vi "Measurement UI.vi"() -> ()   [LabVIEW 2021, in "start-up UI.lvlib"]
uses:
  start-up UI.lvlib
panel:
  in  "Meas Graphs":enum32{"LED V-I Characteristics"}(tab)
  out "LEDInputGraph":cluster{"Value":dbl[], "Value":dbl[]}(graph)
  out "LEDOutputGraph":cluster{dbl[], dbl[]}(graph)
  in  "MeasConfigurations":T1(tab)=enum."Source Config"
  in  "LED current (Io)":dbl=1.0 caption="OUTPUT CURRENT (Io)" format="%.3pA"
  in  "Cumulative forward voltage (Vf)":dbl=1.0 caption="FORWARD VOLTAGE (Vf)" format="%.3fV"
  in  "LED voltage (Vo)":dbl=1.0 caption="OUTPUT VOLTAGE (Vo)" format="%.3fV"
  in  "Source delay":dbl=0.005 caption="SOURCE DELAY" format="%.3ps"
  in  "DUT setup time":dbl=1.0 caption="DUT SETUP TIME" format="%.3ps"
  in  "Aperture time":dbl=0.005 caption="APERTURE TIME" format="%.3ps"
  in  "Source current limit":dbl=14.0 caption="CURRENT LIMIT" format="%#_6pA"
  in  "PPSResourceName":refnum<k15> caption="RESOURCE NAME"
  in  "Source stop voltage":dbl=14.0 caption="VOLTAGE STOP LEVEL" format="%#_6pV"
  in  "Source sense":i32(ring)=1009 caption="SENSE" items=["Local"=1008, "Remote"=1009]
  in  "Source maximum power":dbl=20.0 caption="MAXIMUM POWER" format="%#_6pW"
  in  "Source start voltage":dbl=6.0 caption="VOLTAGE START LEVEL" format="%#_6pV"
  in  "Source voltage sweep points":i32=4 caption="NO. OF POINTS"
  in  "DUT current limit":dbl=6.0 caption="DUT CURRENT LIMIT" format="%#_6pA"
  in  "Load current range":string(combo) caption="CURRENT LIMIT RANGE"
  in  "Load voltage limit":dbl caption="VOLTAGE  LIMIT" format="%#_6pV"
  in  "Load voltage level range":dbl=6.0 caption="VOLTAGE LEVEL RANGE" format="%#_6pV"
  in  "Load sense":i32(ring)=1009 caption="SENSE" items=["Local"=1008, "Remote"=1009]
  in  "LoadResourceName":refnum<k15> caption="RESOURCE NAME"
  out "Status":string
  in  "Max output resistance":string caption="RESOURCE NAME"
  in  "Load current limit range":string caption="RESOURCE NAME"
  out "Load current":dbl[](array[numeric])
  out "Source current":dbl[](array[numeric])
  out "Load voltages":dbl[](array[numeric])
  out "Source voltages":dbl[](array[numeric])
  in  "Source resource name":string caption="RESOURCE NAME"
  in  "Load resource name":string caption="RESOURCE NAME"
  # "V(in) vs I(in)"
  # "Iin vs Vin"
  # "Iout vs Vout"
  # "Emulated LED Configuration"
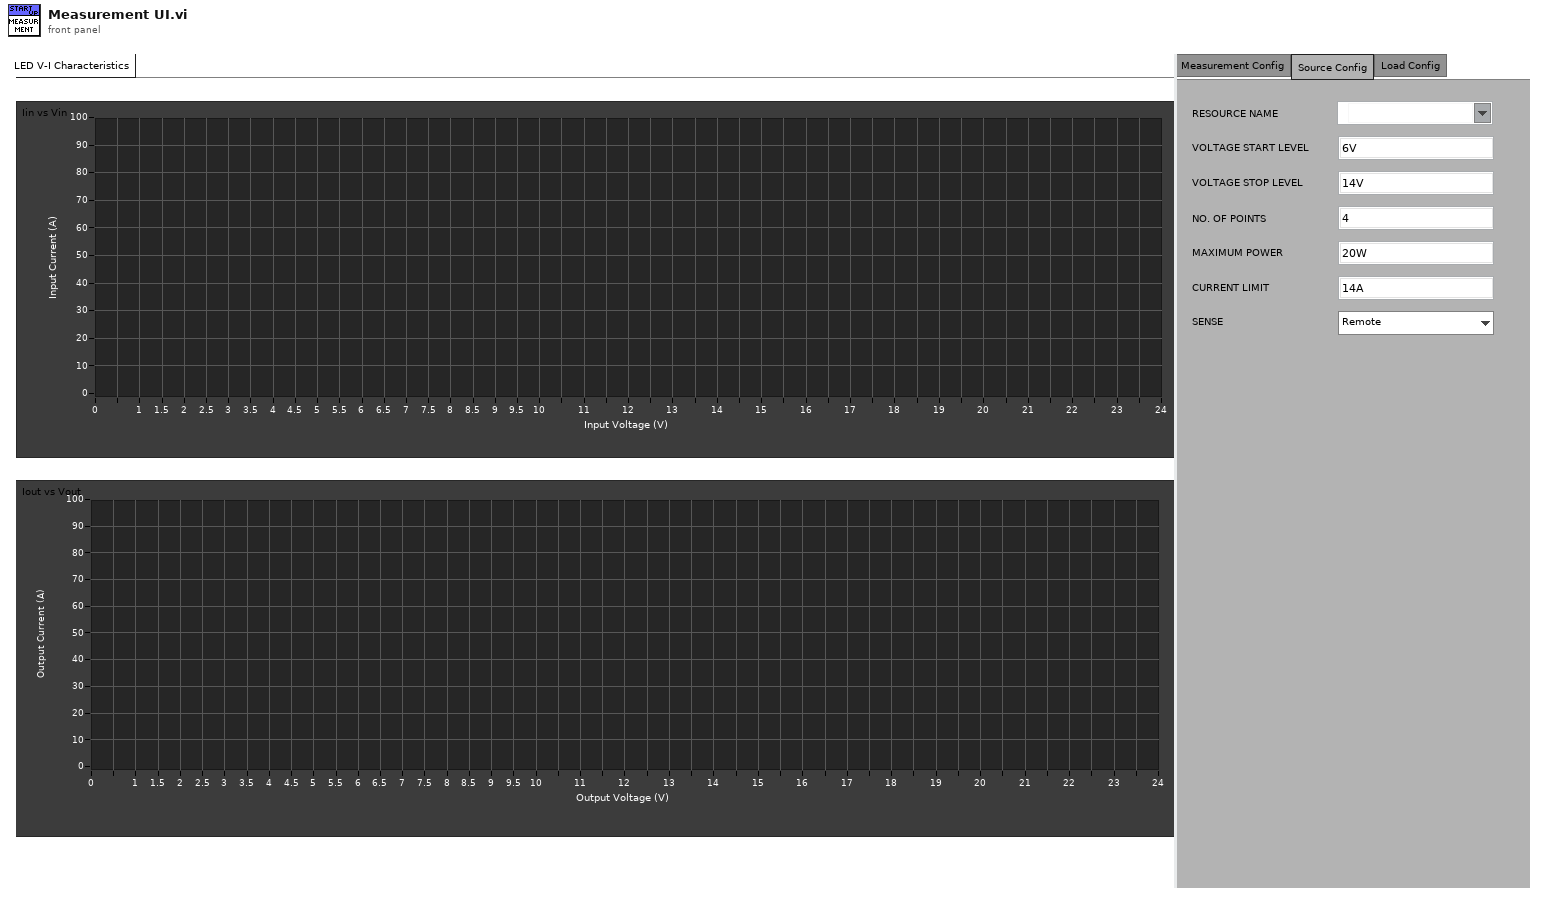
[diagram p1: front panel]
types:
  T1 = enum32{"Measurement Config", "Source Config", "Load Config", "Hidden Controls"}
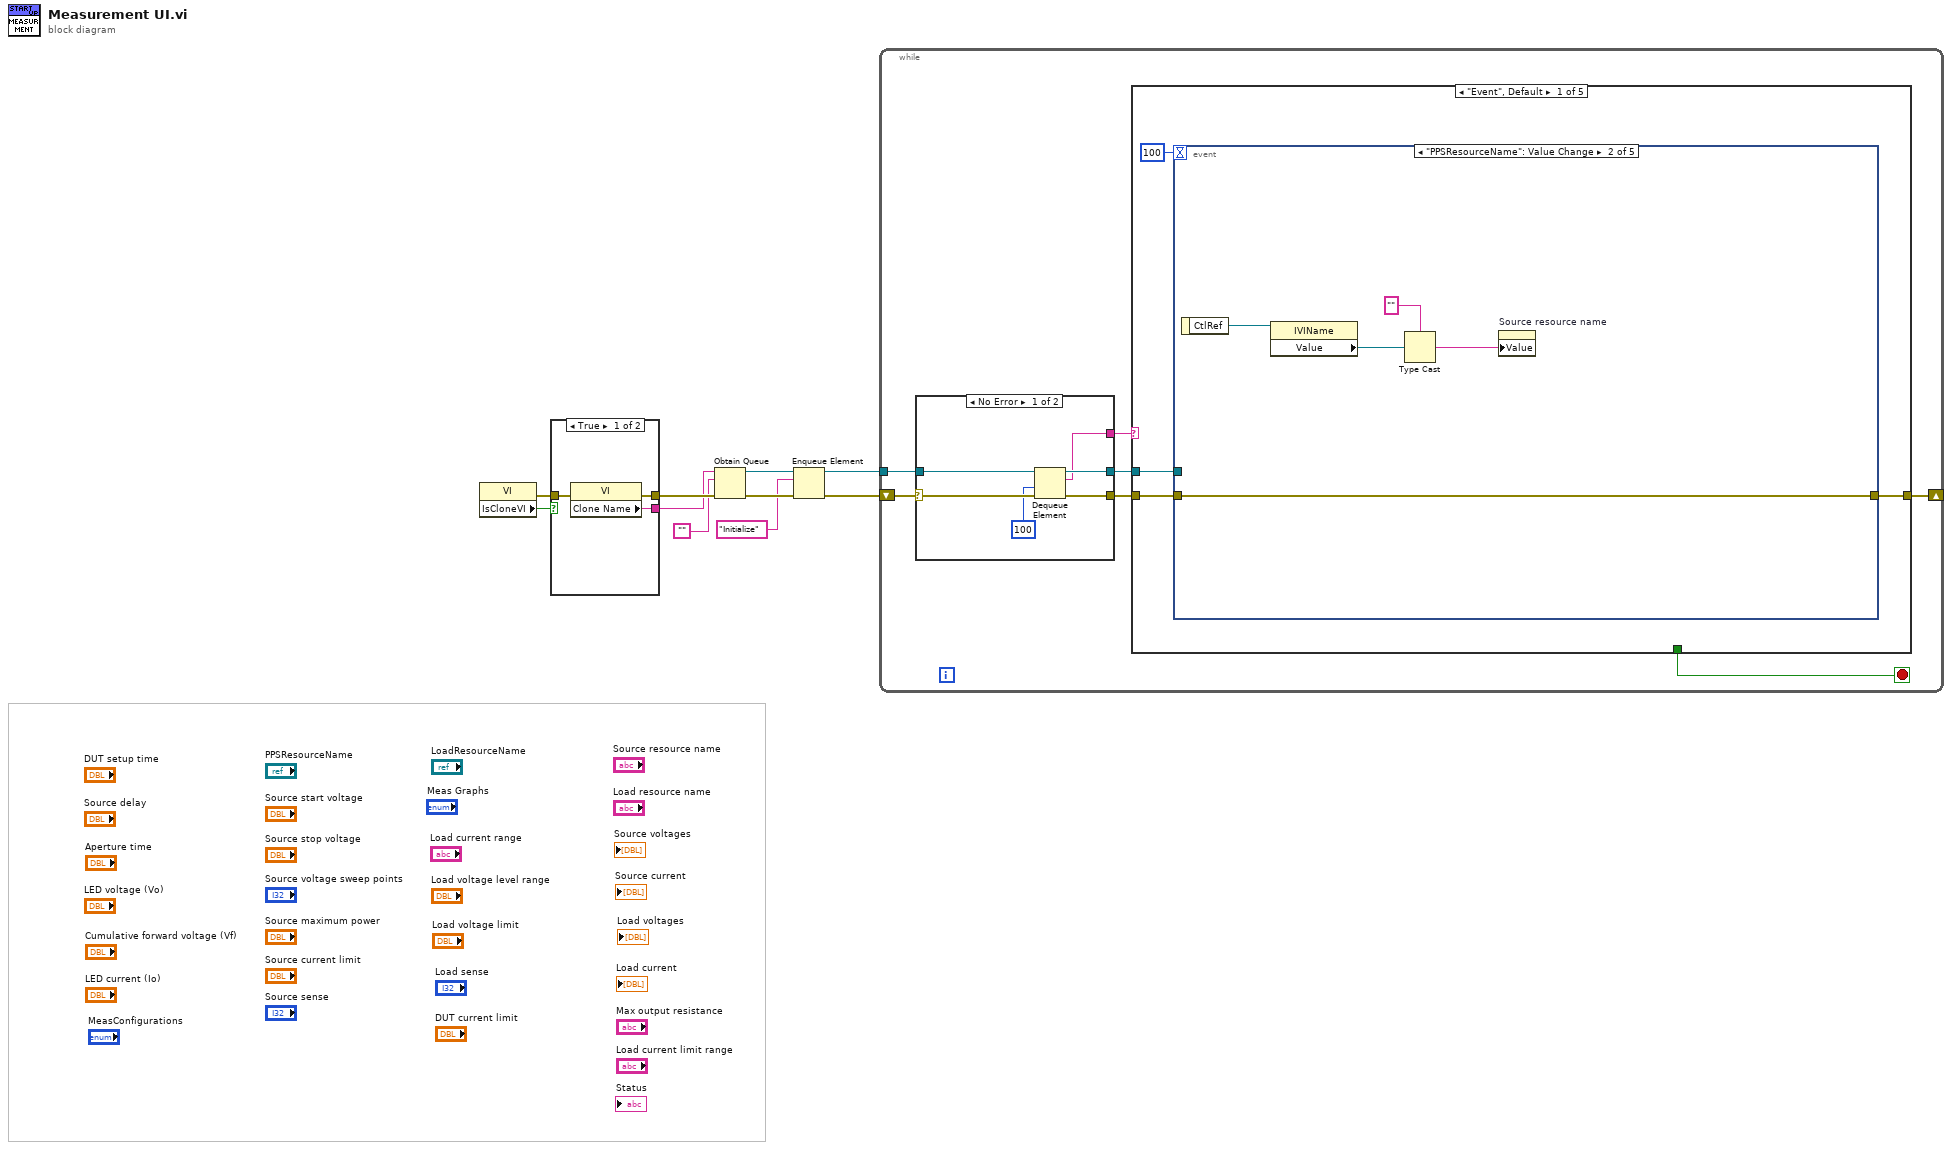
[diagram p0: block diagram]
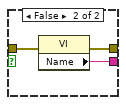
[diagram p2: hidden frame]
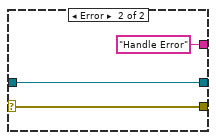
[diagram p3: hidden frame]
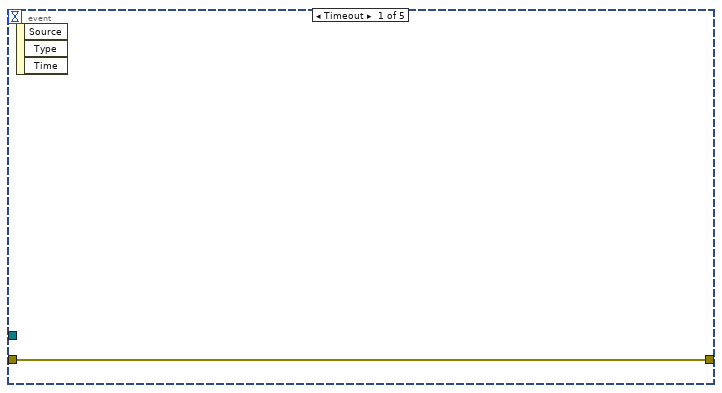
[diagram p4: hidden frame]
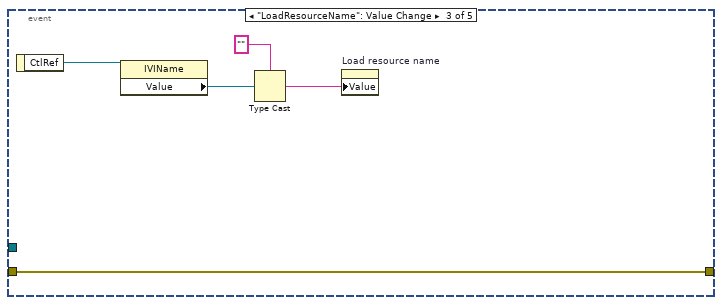
[diagram p5: hidden frame]
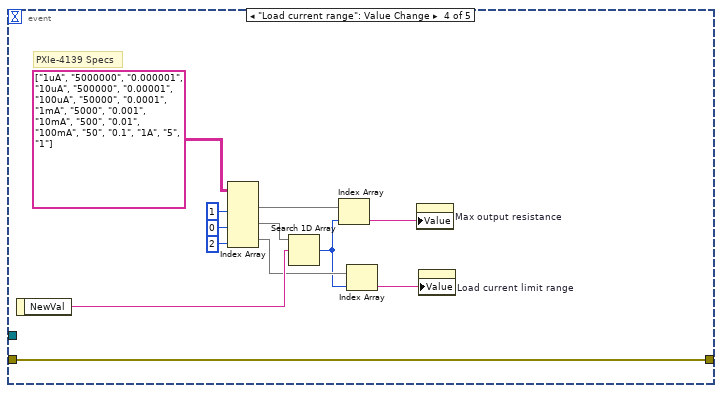
[diagram p6: hidden frame]
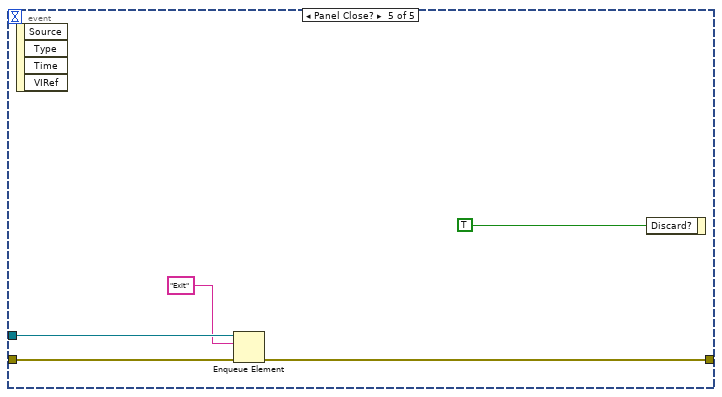
[diagram p7: hidden frame]
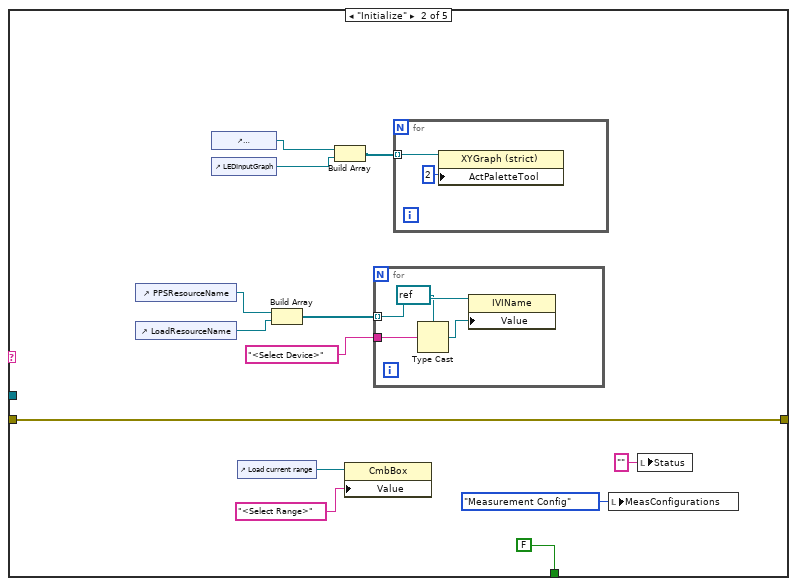
[diagram p8: hidden frame]
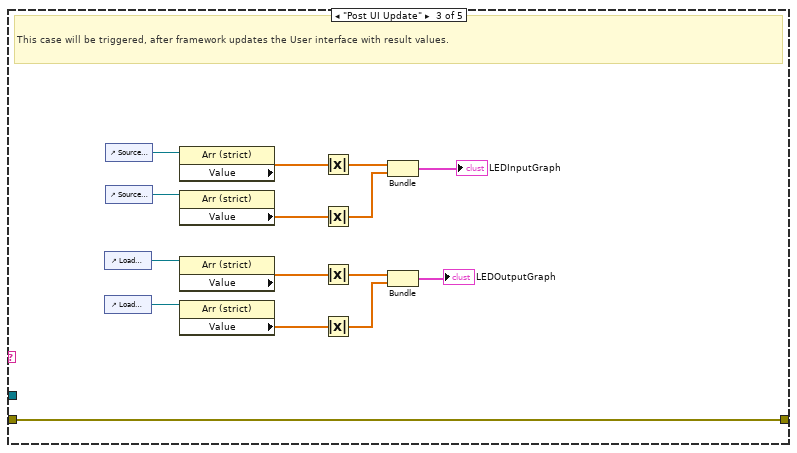
[diagram p9: hidden frame]
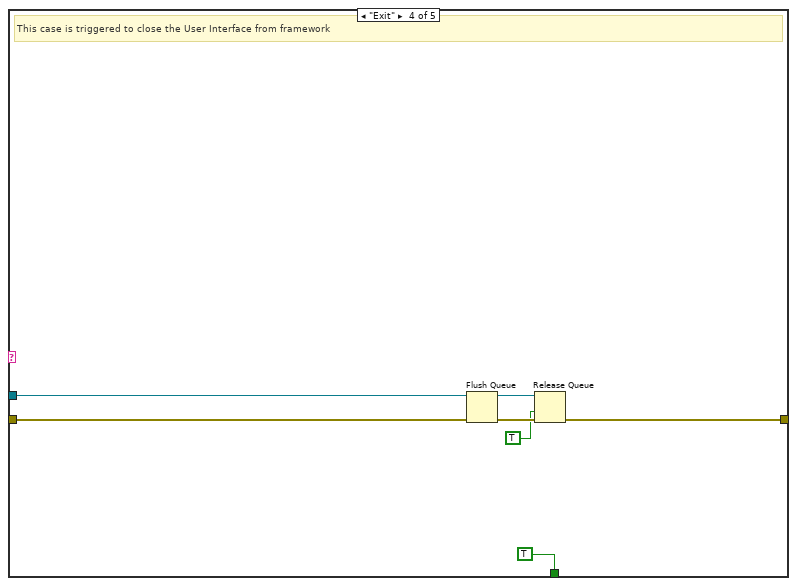
[diagram p10: hidden frame]
diagram:
  n1 = property class="VI"() -> (error out=w1:errorcluster, "IsCloneVI"=w2:bool)  [unwired: 2 in, 1 out]
  n2 = case shown="True" w2 {
    tunnel: [w13 w16] -> w10
    tunnel: [w12 w15] -> w9
    tunnel: w1 -> [w11 w14]
    frame True {
      n3 = property class="VI"(error in=w11) -> (error out=w13:errorcluster, "Clone Name"=w12:string)  [unwired: 1 in, 1 out]
    }
    frame False {
      n4 = property class="VI"(error in=w14) -> (error out=w16:errorcluster, "Name"=w15:string)  [unwired: 1 in, 1 out]
    }
  }
  n5 = Obtain Queue(name (unnamed)=w9, element data type="", error in (no error)=w10) -> (queue out=w6:refnum<queue>, error out=w8:errorcluster)  [unwired: 2 in, 1 out]
  n6 = Enqueue Element(queue=w6, element="Initialize", error in (no error)=w8) -> (queue out=w5:refnum<queue>, error out=w7:errorcluster)  [unwired: 1 in, 1 out]
  n7 = while {
    shift-right: [w18] -> _
    shift-left: w7 -> [w23]
    tunnel: w5 -> [w21]
    stop <- w17 stop-if-true
    n8 = case shown="No Error" w23 {
      selector: w23 -> [w29 w32]
      tunnel: [w28 w32] -> w22
      tunnel: w21 -> [w27 w31]
      tunnel: [w26 w31] -> w20
      tunnel: [w25 "Handle Error"] -> w19
      frame No Error {
        n9 = Dequeue Element(queue=w27, timeout in ms (-1)=100, error in (no error)=w29) -> (queue out=w26:refnum<queue>, element=w25:string, error out=w28:errorcluster)  [unwired: 1 out]
      }
      frame Error {
      }
    }
    n10 = case shown="\"Event\", Default" w19 {
      tunnel: w22 -> [w35 w77 w98 w105 w106]
      tunnel: w20 -> [w33 _ _ w103 _]
      tunnel: [w36 w77 w98 w100 w106] -> w18
      tunnel: [_ FALSE _ TRUE _] -> w17
      frame "Event", Default {
        n11 = event shown="[1] \"PPSResourceName\": Value Change" {
          selector: _ -> [_ _ _ _ _]
          dyn-events: _ -> [_ _ _ _ _]
          timeout: 100 -> [_ _ _ _ _]
          tunnel: [w37 w38 w43 w54 w62] -> w36
          tunnel: w35 -> [w37 w38 w43 w54 w63]
          tunnel: w33 -> [_ _ _ _ w61]
          event Timeout {
            n12 = event-data() -> ()  [unwired: 1 in, 3 out]
          }
          event "PPSResourceName": Value Change {
            n13 = event-data() -> ("CtlRef"=w42:refnum<vi>)  [unwired: 1 in]
            n14 = property class="IVIName"(reference=w42) -> ("Value"=w40:refnum<k15>)  [unwired: 1 in, 2 out]
            n15 = Type Cast(type="", x=w40) -> (*(type *) &x=w41:string)
            n16 = property on="Source resource name" class="Str"("Value"=w41) -> ()  [unwired: 2 in, 2 out]
          }
          event "LoadResourceName": Value Change {
            n17 = event-data() -> ("CtlRef"=w45:refnum<vi>)  [unwired: 1 in]
            n18 = property class="IVIName"(reference=w45) -> ("Value"=w47:refnum<k15>)  [unwired: 1 in, 2 out]
            n19 = Type Cast(type="", x=w47) -> (*(type *) &x=w44:string)
            n20 = property on="Load resource name" class="Str"("Value"=w44) -> ()  [unwired: 2 in, 2 out]
          }
          event "Load current range": Value Change {
            # "PXIe-4139 Specs"
            n21 = event-data() -> ("NewVal"=w57:string)  [unwired: 1 in]
            n22 = Index Array(array=string[][] [["1uA", "5000000", "0.000001"], ["10uA", "500000", "0.00001"], ["100uA", "50000", "0.0001"], ["1mA", "5000", "0.001"], ["10mA", "500", "0.01"], ["100mA", "50", "0.1"], ["1A", "5", "1"]], index (col) #1=1 ("disabled index (col)"), index (col) #2=0 ("index (col)"), index (col) #3=2 ("index (col)")) -> (element #1=w55:string[], element #2=w50:string[], element #3=w51:string[])  [unwired: 3 in]
            n23 = Search 1D Array(1D array=w50, element=w57) -> (index of element=w49:i32)  [unwired: 1 in]
            n24 = Index Array(array=w55, index=w49) -> (element=w53:string)
            n25 = Index Array(array=w51, index=w49) -> (element=w48:string)
            n26 = property on="Max output resistance" class="Str"("Value"=w53) -> ()  [unwired: 2 in, 2 out]
            n27 = property on="Load current limit range" class="Str"("Value"=w48) -> ()  [unwired: 2 in, 2 out]
          }
          event Panel Close? {
            n28 = event-data() -> ()  [unwired: 1 in, 4 out]
            n29 = Enqueue Element(queue=w61, element="Exit", error in (no error)=w63) -> (error out=w62:errorcluster)  [unwired: 1 in, 2 out]
            n30 = event-data("Discard?"=TRUE) -> ()  [unwired: 1 in, 1 out]
          }
        }
      }
      frame "Initialize" {
        n31 = control-ref of="PPSResourceName"() -> (w72:refnum<vi>)
        n32 = control-ref of="LoadResourceName"() -> (w71:refnum<vi>)
        n33 = control-ref of="LEDOutputGraph"() -> (w74:refnum<vi>)
        n34 = control-ref of="LEDInputGraph"() -> (w73:refnum<vi>)
        n35 = control-ref of="Load current range"() -> (w68:refnum<vi>)
        n36 = Build Array(w72, w71) -> (w70:refnum<vi>[])
        n37 = Build Array(w74, w73) -> (w75:refnum<vi>[])
        n38 = property class="CmbBox"(reference=w68, "Value"="<Select Range>") -> ()  [unwired: 1 in, 2 out]
        n39 = for {
          tunnel: w70 -> [w81] mode=indexing
          tunnel: "<Select Device>" -> [w80]
          n40 = Type Cast(type=refnum<k15> refnum ("Value"), x=w80) -> (*(type *) &x=w78:refnum<k15>)
          n41 = property class="IVIName"(reference=w81, "Value"=w78) -> ()  [unwired: 1 in, 2 out]
        }
        n42 = for {
          tunnel: w75 -> [w82] mode=indexing
          n43 = property class="XYGraph (strict)"(reference=w82, "ActPaletteTool"=2 ("Palette:Active Tool")) -> ()  [unwired: 1 in, 2 out]
        }
        n44 = local write "MeasConfigurations"(T1."Measurement Config" ("MeasConfigurations")) -> ()
        n45 = local write "Status"("" ("Status")) -> ()
      }
      frame "Post UI Update" {
        # "This case will be triggered, after framework updates the User interface with result values."
        n46 = control-ref of="Load voltages"() -> (w87:refnum<vi>)
        n47 = control-ref of="Load current"() -> (w86:refnum<vi>)
        n48 = control-ref of="Source voltages"() -> (w97:refnum<vi>)
        n49 = control-ref of="Source current"() -> (w96:refnum<vi>)
        n50 = property class="Arr (strict)"(reference=w97) -> ("Value"=w95:dbl[])  [unwired: 1 in, 2 out]
        n51 = property class="Arr (strict)"(reference=w96) -> ("Value"=w94:dbl[])  [unwired: 1 in, 2 out]
        n52 = property class="Arr (strict)"(reference=w87) -> ("Value"=w88:dbl[])  [unwired: 1 in, 2 out]
        n53 = property class="Arr (strict)"(reference=w86) -> ("Value"=w89:dbl[])  [unwired: 1 in, 2 out]
        n54 = Absolute Value(x=w95) -> (abs(x)=w93:dbl[])
        n55 = Absolute Value(x=w94) -> (abs(x)=w92:dbl[])
        n56 = Absolute Value(x=w88) -> (abs(x)=w90:dbl[])
        n57 = Absolute Value(x=w89) -> (abs(x)=w91:dbl[])
        n58 = Bundle(w93, w92) -> (→"LEDInputGraph":cluster{dbl[], dbl[]})  [unwired: 1 in]
        n59 = Bundle(w90, w91) -> (→"LEDOutputGraph":cluster{dbl[], dbl[]})  [unwired: 1 in]
      }
      frame "Exit" {
        # "This case is triggered to close the User Interface from framework"
        n60 = Flush Queue(queue=w103, error in (no error)=w105) -> (queue out=w102:refnum<queue>, error out=w101:errorcluster)  [unwired: 1 out]
        n61 = Release Queue(queue=w102, force destroy? (F)=TRUE, error in (no error)=w101) -> (error out=w100:errorcluster)  [unwired: 2 out]
      }
      frame "Handle Error" {
      }
    }
  }
